vi "Main.vi"() -> ()   [LabVIEW 2018]
uses:
  S4GUI/S4GUI.lvclass
  Interface/Interface.lvclass/Interface.ctl
  S4GUI/S4GUI.lvclass/S4GUI.ctl
  Instrument/Instrument.lvclass/Instrument.ctl
  Device/Optics/Optics.lvclass/Optics.ctl
  Device/Optics/Opt_Selector/Opt_Selector.lvclass
  C:/Users/observer/Desktop/Sparc4GUI/SPARC4_GUI/Device/Optics/Optics.lvclass
  Instrument/Instrument.lvclass
  Acquisition/Acquisition.lvclass
  Channel/Channel.lvclass
  Interface/Interface.lvclass
  StateMachine/State Machine.lvclass
  Device/Optics/Optics.lvclass
panel:
  in  "Set Waveplate":bool
  in  "Calibrator Selector":u16(ring) items=["OFF", "Polarizer", "Depolarizer"]
  in  "Waveplate Selector":u16(ring) items=["OFF", "Lambda/2", "Lambda/4"]
  in  "START ch1":bool
  in  "Exptime ch1":dbl
  in  "exit":bool
  in  "S4GUI.lvclass":refnum<class "S4GUI.lvclass">
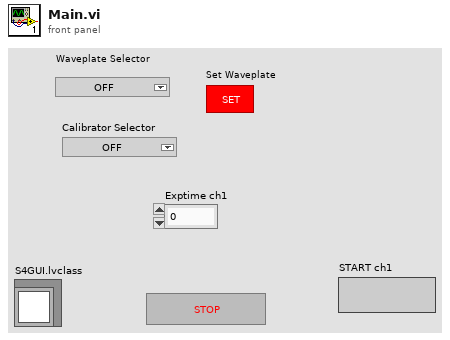
[diagram p1: front panel]
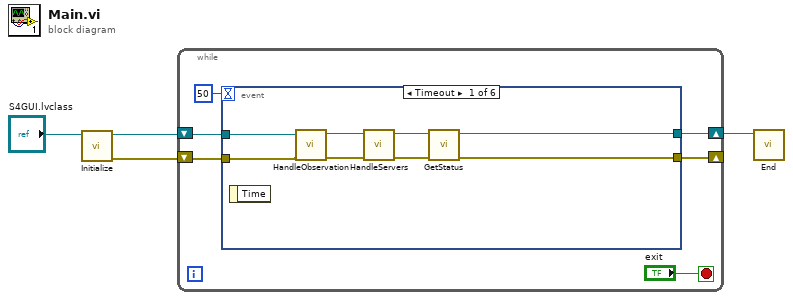
[diagram p0: block diagram]
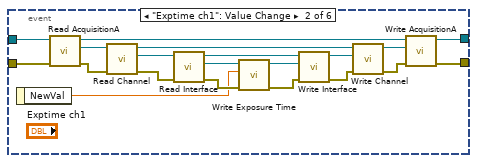
[diagram p2: hidden frame]
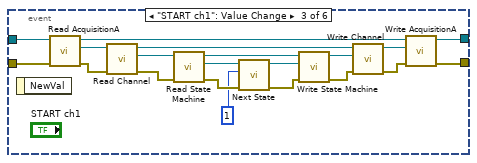
[diagram p3: hidden frame]
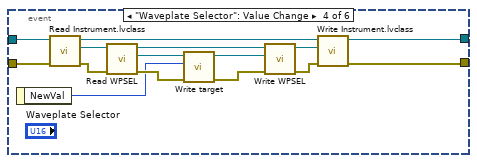
[diagram p4: hidden frame]
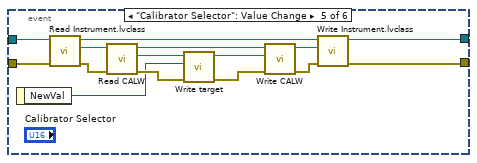
[diagram p5: hidden frame]
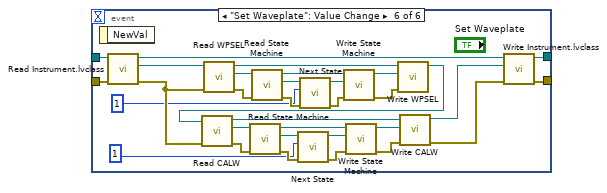
[diagram p6: hidden frame]
diagram:
  n1 = call-dynamic "Initialize.vi"("S4ACS_GUI in"="S4GUI.lvclass") -> ("error out"=w1:errorcluster, "S4ACS_GUI out"=w3:refnum<class "S4GUI.lvclass">)  [unwired: 9 in]
  n2 = while {
    shift-right: [w7] -> w2
    shift-left: w3 -> [w8]
    shift-right: [w5] -> _
    shift-left: w1 -> [w6]
    stop <- "exit" stop-if-true
    n3 = event shown="[0] Timeout" {
      selector: _ -> [_ _ _ _ _ _]
      dyn-events: _ -> [_ _ _ _ _ _]
      timeout: 50 -> [_ _ _ _ _ _]
      tunnel: w8 -> [w18 w23 w43 w65 w80 w109]
      tunnel: [w15 w21 w41 w63 w78 w107] -> w7
      tunnel: w6 -> [w14 w22 w42 w64 w79 w108]
      tunnel: [w11 w20 w40 w62 w77 w106] -> w5
      event Timeout {
        n4 = event-data() -> ()  [unwired: 1 in, 1 out]
        n5 = call-dynamic "HandleObservation.vi"("error in (no error)"=w14, "S4ACS_GUI in"=w18) -> ("error out"=w13:errorcluster, "S4ACS_GUI out"=w17:refnum<class "S4GUI.lvclass">)  [unwired: 8 in]
        n6 = call-dynamic "HandleServers.vi"("error in (no error)"=w13, "S4ACS_GUI in"=w17) -> ("error out"=w12:errorcluster, "S4ACS_GUI out"=w16:refnum<class "S4GUI.lvclass">)  [unwired: 8 in]
        n7 = call-dynamic "GetStatus.vi"("error in (no error)"=w12, "S4ACS_GUI in"=w16) -> ("error out"=w11:errorcluster, "S4ACS_GUI out"=w15:refnum<class "S4GUI.lvclass">)  [unwired: 6 in, 2 out]
      }
      event "Exptime ch1": Value Change {
        n8 = event-data() -> ("NewVal"=w19:dbl)  [unwired: 1 in]
        n9 = call-dynamic "Read AcquisitionA.vi"("error in (no error)"=w22, "S4ACS_GUI in"=w23) -> ("error out"=w25:errorcluster, "Acquisition.lvclass"=w24:refnum<class "Acquisition.lvclass">, "S4ACS_GUI out"=w27:refnum<class "S4GUI.lvclass">)  [unwired: 7 in]
        n10 = call-dynamic "Read Channel.vi"("error in (no error)"=w25, "Acquisition in"=w24) -> ("error out"=w36:errorcluster, "Channel.lvclass"=w35:refnum<class "Channel.lvclass">, "Acquisition out"=w34:refnum<class "Acquisition.lvclass">)  [unwired: 7 in]
        n11 = call-dynamic "Read Interface.vi"("error in (no error)"=w36, "Channel in"=w35) -> ("error out"=w30:errorcluster, "Interface.lvclass"=w29:refnum<class "Interface.lvclass">, "Channel out"=w31:refnum<class "Channel.lvclass">)  [unwired: 7 in]
        n12 = call "Write Exposure Time.vi"("error in (no error)"=w30, "Exposure Time"=w19, "Interface in"=w29) -> ("error out"=w38:errorcluster, "Interface out"=w37:refnum<class "Interface.lvclass">)  [unwired: 7 in]
        n13 = call-dynamic "Write Interface.vi"("error in (no error)"=w38, "Interface.lvclass"=w37, "Channel in"=w31) -> ("error out"=w32:errorcluster, "Channel out"=w33:refnum<class "Channel.lvclass">)  [unwired: 7 in]
        n14 = call-dynamic "Write Channel.vi"("error in (no error)"=w32, "Channel.lvclass"=w33, "Acquisition in"=w34) -> ("error out"=w28:errorcluster, "Acquisition out"=w26:refnum<class "Acquisition.lvclass">)  [unwired: 7 in]
        n15 = call-dynamic "Write AcquisitionA.vi"("error in (no error)"=w28, "Acquisition.lvclass"=w26, "S4ACS_GUI in"=w27) -> ("error out"=w20:errorcluster, "S4ACS_GUI out"=w21:refnum<class "S4GUI.lvclass">)  [unwired: 7 in]
      }
      event "START ch1": Value Change {
        n16 = event-data() -> ()  [unwired: 1 in, 1 out]
        n17 = call-dynamic "Read AcquisitionA.vi"("error in (no error)"=w42, "S4ACS_GUI in"=w43) -> ("error out"=w45:errorcluster, "Acquisition.lvclass"=w44:refnum<class "Acquisition.lvclass">, "S4ACS_GUI out"=w47:refnum<class "S4GUI.lvclass">)  [unwired: 7 in]
        n18 = call-dynamic "Read Channel.vi"("error in (no error)"=w45, "Acquisition in"=w44) -> ("error out"=w56:errorcluster, "Channel.lvclass"=w55:refnum<class "Channel.lvclass">, "Acquisition out"=w54:refnum<class "Acquisition.lvclass">)  [unwired: 7 in]
        n19 = call-dynamic "Read State Machine.vi"("error in (no error)"=w56, "Device in"=w55) -> ("error out"=w50:errorcluster, "State Machine.lvclass"=w49:refnum<class "State Machine.lvclass">, "Device out"=w51:refnum<class "Channel.lvclass">)  [unwired: 7 in]
        n20 = call "Next State.vi"("error in (no error)"=w50, "New_State"=1, "State Machine in"=w49) -> ("error out"=w58:errorcluster, "State Machine out"=w57:refnum<class "State Machine.lvclass">)  [unwired: 7 in]
        n21 = call-dynamic "Write State Machine.vi"("error in (no error)"=w58, "State Machine.lvclass"=w57, "Device in"=w51) -> ("error out"=w52:errorcluster, "Device out"=w53:refnum<class "Channel.lvclass">)  [unwired: 7 in]
        n22 = call-dynamic "Write Channel.vi"("error in (no error)"=w52, "Channel.lvclass"=w53, "Acquisition in"=w54) -> ("error out"=w48:errorcluster, "Acquisition out"=w46:refnum<class "Acquisition.lvclass">)  [unwired: 7 in]
        n23 = call-dynamic "Write AcquisitionA.vi"("error in (no error)"=w48, "Acquisition.lvclass"=w46, "S4ACS_GUI in"=w47) -> ("error out"=w40:errorcluster, "S4ACS_GUI out"=w41:refnum<class "S4GUI.lvclass">)  [unwired: 7 in]
      }
      event "Waveplate Selector": Value Change {
        n24 = event-data() -> ("NewVal"=w61:u16)  [unwired: 1 in]
        n25 = call "Read Instrument.lvclass.vi"("error in (no error)"=w64, "S4ACS_GUI in"=w65) -> ("error out"=w67:errorcluster, "Instrument.lvclass"=w66:refnum<class "Instrument.lvclass">, "S4ACS_GUI out"=w69:refnum<class "S4GUI.lvclass">)  [unwired: 7 in]
        n26 = call "Read WPSEL.vi"("error in (no error)"=w67, "Instrument in"=w66) -> ("error out"=w73:errorcluster, "Opt_Selector.lvclass"=w72:refnum<class "Opt_Selector.lvclass">, "Instrument out"=w71:refnum<class "Instrument.lvclass">)  [unwired: 7 in]
        n27 = call "Write target.vi"("error in (no error)"=w73, "target"=w61, "Optics in"=w72) -> ("error out"=w60:errorcluster, "Optics out"=w59:refnum<class "Opt_Selector.lvclass">)  [unwired: 7 in]
        n28 = call "Write WPSEL.vi"("error in (no error)"=w60, "Opt_Selector.lvclass"=w59, "Instrument in"=w71) -> ("error out"=w70:errorcluster, "Instrument out"=w68:refnum<class "Instrument.lvclass">)  [unwired: 7 in]
        n29 = call "Write Instrument.lvclass.vi"("error in (no error)"=w70, "Instrument.lvclass"=w68, "S4ACS_GUI in"=w69) -> ("error out"=w62:errorcluster, "S4ACS_GUI out"=w63:refnum<class "S4GUI.lvclass">)  [unwired: 7 in]
      }
      event "Calibrator Selector": Value Change {
        n30 = event-data() -> ("NewVal"=w76:u16)  [unwired: 1 in]
        n31 = call "Read Instrument.lvclass.vi"("error in (no error)"=w79, "S4ACS_GUI in"=w80) -> ("error out"=w82:errorcluster, "Instrument.lvclass"=w81:refnum<class "Instrument.lvclass">, "S4ACS_GUI out"=w84:refnum<class "S4GUI.lvclass">)  [unwired: 7 in]
        n32 = call "Read CALW.vi"("error in (no error)"=w82, "Instrument in"=w81) -> ("error out"=w88:errorcluster, "Opt_Selector.lvclass"=w87:refnum<class "Opt_Selector.lvclass">, "Instrument out"=w86:refnum<class "Instrument.lvclass">)  [unwired: 7 in]
        n33 = call "Write target.vi"("error in (no error)"=w88, "target"=w76, "Optics in"=w87) -> ("error out"=w75:errorcluster, "Optics out"=w74:refnum<class "Opt_Selector.lvclass">)  [unwired: 7 in]
        n34 = call "Write CALW.vi"("error in (no error)"=w75, "Opt_Selector.lvclass"=w74, "Instrument in"=w86) -> ("error out"=w85:errorcluster, "Instrument out"=w83:refnum<class "Instrument.lvclass">)  [unwired: 7 in]
        n35 = call "Write Instrument.lvclass.vi"("error in (no error)"=w85, "Instrument.lvclass"=w83, "S4ACS_GUI in"=w84) -> ("error out"=w77:errorcluster, "S4ACS_GUI out"=w78:refnum<class "S4GUI.lvclass">)  [unwired: 7 in]
      }
      event "Set Waveplate": Value Change {
        n36 = event-data() -> ()  [unwired: 1 in, 1 out]
        n37 = call "Read Instrument.lvclass.vi"("error in (no error)"=w108, "S4ACS_GUI in"=w109) -> ("error out"=w95:errorcluster, "Instrument.lvclass"=w94:refnum<class "Instrument.lvclass">, "S4ACS_GUI out"=w110:refnum<class "S4GUI.lvclass">)  [unwired: 7 in]
        n38 = call "Read WPSEL.vi"("error in (no error)"=w95, "Instrument in"=w94) -> ("error out"=w118:errorcluster, "Opt_Selector.lvclass"=w117:refnum<class "Opt_Selector.lvclass">, "Instrument out"=w116:refnum<class "Instrument.lvclass">)  [unwired: 7 in]
        n39 = call-dynamic "Read State Machine.vi"("error in (no error)"=w118, "Device in"=w117) -> ("error out"=w112:errorcluster, "State Machine.lvclass"=w111:refnum<class "State Machine.lvclass">, "Device out"=w113:refnum<class "Opt_Selector.lvclass">)  [unwired: 7 in]
        n40 = call "Next State.vi"("error in (no error)"=w112, "New_State"=1, "State Machine in"=w111) -> ("error out"=w120:errorcluster, "State Machine out"=w119:refnum<class "State Machine.lvclass">)  [unwired: 7 in]
        n41 = call-dynamic "Write State Machine.vi"("error in (no error)"=w120, "State Machine.lvclass"=w119, "Device in"=w113) -> ("error out"=w114:errorcluster, "Device out"=w115:refnum<class "Opt_Selector.lvclass">)  [unwired: 7 in]
        n42 = call "Write WPSEL.vi"("error in (no error)"=w114, "Opt_Selector.lvclass"=w115, "Instrument in"=w116) -> ("Instrument out"=w91:refnum<class "Instrument.lvclass">)  [unwired: 7 in, 1 out]
        n43 = call "Read CALW.vi"("error in (no error)"=w95, "Instrument in"=w91) -> ("error out"=w103:errorcluster, "Opt_Selector.lvclass"=w102:refnum<class "Opt_Selector.lvclass">, "Instrument out"=w90:refnum<class "Instrument.lvclass">)  [unwired: 7 in]
        n44 = call-dynamic "Read State Machine.vi"("error in (no error)"=w103, "Device in"=w102) -> ("error out"=w98:errorcluster, "State Machine.lvclass"=w97:refnum<class "State Machine.lvclass">, "Device out"=w99:refnum<class "Opt_Selector.lvclass">)  [unwired: 7 in]
        n45 = call "Next State.vi"("error in (no error)"=w98, "New_State"=1, "State Machine in"=w97) -> ("error out"=w105:errorcluster, "State Machine out"=w104:refnum<class "State Machine.lvclass">)  [unwired: 7 in]
        n46 = call-dynamic "Write State Machine.vi"("error in (no error)"=w105, "State Machine.lvclass"=w104, "Device in"=w99) -> ("error out"=w100:errorcluster, "Device out"=w101:refnum<class "Opt_Selector.lvclass">)  [unwired: 7 in]
        n47 = call "Write CALW.vi"("error in (no error)"=w100, "Opt_Selector.lvclass"=w101, "Instrument in"=w90) -> ("error out"=w92:errorcluster, "Instrument out"=w93:refnum<class "Instrument.lvclass">)  [unwired: 7 in]
        n48 = call "Write Instrument.lvclass.vi"("error in (no error)"=w92, "Instrument.lvclass"=w93, "S4ACS_GUI in"=w110) -> ("error out"=w106:errorcluster, "S4ACS_GUI out"=w107:refnum<class "S4GUI.lvclass">)  [unwired: 7 in]
      }
    }
  }
  n49 = call-dynamic "End.vi"("S4ACS_GUI in"=w2) -> ()  [unwired: 9 in, 2 out]
